vi "Example1.1-Waveform Generator.vi"() -> ()   [LabVIEW 2013]
panel:
  out "Waveform Graph":dynamicdata(graph)=[{"t0"=timestamp(2926.7000000000003 s since 1904-01-01), "dt"=0.0001, "Y"=array[1000 elements], "attributes"=variant("NI_ChannelName"=variant(string "Sine"), "NI_ExpIsRelativeTime"=variant(bool TRUE), "NI_ExpStartTimeStamp"=variant(timestamp timestamp(3695299042.4811053 s since 1904-01-01)), "NI_ExpTimeStamp"=variant(timestamp timestamp(3695301969.181105 s since 1904-01-01)), "NI_ExpXDimension"=variant(string "t"))}]
  in  "初相位":dbl caption="Phase"
  in  "频率":dbl=100.0 caption="Frequency"
  in  "幅度":dbl=1.0 caption="Amplitude"
  in  "信号类型":string(combo)="Sine"
  in  "stop":bool
  # "波形信号发生器"
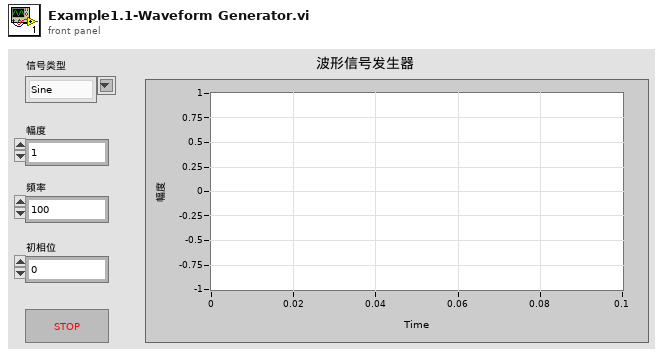
[diagram p1: front panel]
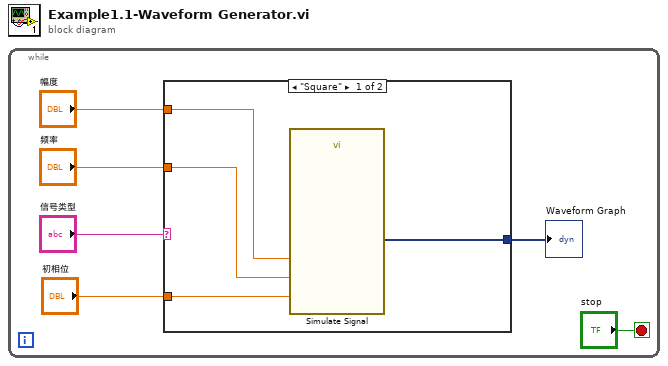
[diagram p0: block diagram]
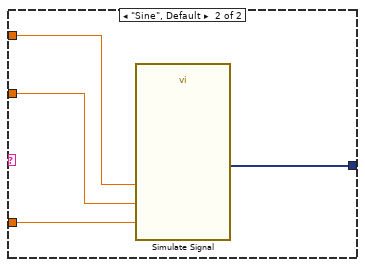
[diagram p2: hidden frame]
diagram:
  n1 = while {
    stop <- "stop" stop-if-true
    n2 = case shown="\"Square\"" "信号类型" {
      tunnel: "幅度" -> [w8 w14]
      tunnel: "频率" -> [w7 w13]
      tunnel: "初相位" -> [w9 w12]
      tunnel: [w10 w11] -> w1
      frame "Square" {
        n3 = call "Simulate Signal"("Frequency"=w7, "Amplitude"=w8, "Phase"=w9) -> ("Square"=w10:dynamicdata)  [unwired: 11 in, 1 out]
      }
      frame "Sine", Default {
        n4 = call "Simulate Signal"("Frequency"=w13, "Amplitude"=w14, "Phase"=w12) -> ("Sine"=w11:dynamicdata)  [unwired: 11 in, 1 out]
      }
    }
    "Waveform Graph" <- w1
  }
